vi "rs3 is advanced mode enabled.vi"(8 "error in (no error)":errorcluster, 11 "device in":u64) -> (0 "error out":errorcluster, 1 "error":u64, 2 "enable?":i32, 3 "device out":u64)   [LabVIEW 2023]
doc: "Queries whether the device is in ADVANCED MODE. If it is not, then it will not be possible to set many of the advanced depth and color settings. \n\nINPUT: \nDev in Input device\n\nOUTPUT:\nEnable? Is it enabled\nerror Error=0 is no error"
panel:
  # "RS3 is Advanced Mode Enabled"
  # "(C) 2017 Intel Corp.,  AGJ"
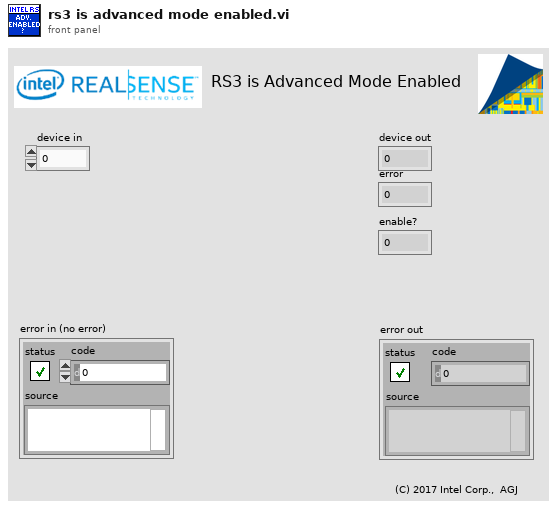
[diagram p1: front panel]
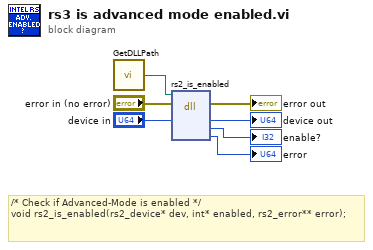
[diagram p0: block diagram]
diagram:
  # "/* Check if Advanced-Mode is enabled */\nvoid rs2_is_enabled(rs2_device* dev, int* enabled, rs2_error** error);"
  n1 = call "GetDLLPath.vi"() -> ("DLL Path"=w1:path)
  n2 = dll-call lib="C:/STEAMSyndicate/RealSenseWrappers/VI Wrappers (add ons) Public/RealSense/realsense2.dll" fn="rs2_is_enabled"(path in=w1, error in="error in (no error)", "device in"="device in") -> (error out=→"error out":errorcluster, "device in"=→"device out":u64, "enable?"=→"enable?":i32, "error"=→"error":u64)  [unwired: 4 in, 1 out]
